vi "NEW数据采集传输系统.vi"() -> ()   [LabVIEW 2016, in "数据传输系统-02.lvlib"]
uses:
  <vilib>/Utility/miscctls.llb/LVPointTypeDef.ctl
  <vilib>/picture/picture.llb/imagedata.ctl
  <vilib>/Utility/config.llb/NI_LVConfig.lvlib
  update/update.lvlib
panel:
  in  "每日自动重发":bool
  in  "串口透传":bool
  in  "共享MN":bool
  out "剖面数据补发":bool
  out "日志信息补发":bool
  out "数据补发":bool
  in  "自动更新":bool
  in  "数据补传":bool caption="确定"
  out "数据库打开失败次数":dbl
  out "与工控通信指示灯":bool
  out "判断数据反馈":enum16{"非严格判断", "严格判断", "不判断"}(ring)
  in  "暂停上传":bool
  in  "配置表":bool caption="确定"
  in  "updateconfiguration":T1={"主机"="27.154.58.30", "用户"="update", "密码"="std23506", "远程路径"="数据传输系统\\平台数据传输系统.exe", "下载文件名"="平台数据传输系统.exe", "软件版本"=""}
  out "标题显示":string
  in  "更新":bool
  in  "系统编码选择框":string(combo)="地表水质量监测"
  out "数据发送通道":enum16{"TCP", "VISA"}(ring)
  in  "baud rate":u32=9600 caption="波特率"
  in  "VISA resource name":refnum<visa-resource-name> caption="VISA资源名称"
  in  "实时数据发送时间间隔/min":i32=1
  in  "数据组合发送":bool
  in  "2011发送":bool
  out "数据发送协议":enum16{"2005-212协议", "2017-212协议"}(ring)=enum."2017-212协议"
  in  "重发时间":T2(ring)
  in  "重发日期":T3(ring)
  in  "开机启动":bool
  in  "每周自动重发":bool=TRUE
  in  "确定":bool
  in  "返回":bool
  in  "PW":string
  in  "MN":string
  in  "PORT":string
  in  "IP":string
  in  "站点设备":string
  in  "站点名称":string
  out "设置超时时间/min":i32=1
  out "状态信息":T4={"1st Error to Convert "=63, "步骤 "=enum."发送数据", "元素"="实时数据", "TCP服务端掉线计数"=0, "TCP掉线时间节点"="2019/05/08 15:24:17"} {"1st Error to Convert" items=["无错误", "参数错误", "内存已满", "超出区域", "文件结束", "文件已打开", "一般文件IO错误", "未找到文件", "文件权限错误", "磁盘已满", "路径副本", "打开过多文件", "未启用", "未找到资源文件", "无法添加资源", "未找到资源", "未找到图像", "图像内存错误", "画笔不存在", "配置错误类型", "配置未找到解析段", "配置解析错误", "配置内存错误", "错误外部代码格式", "错误外部代码偏移量", "外部代码不存在", "空窗口", "销毁窗口错误", "空菜单", "打印已中止", "错误打印记录", "打印驱动程序错误", "打印时窗口错误", "打印时内存错误", "打印对话框错误", "一般打印错误", "无效设备引用句柄", "设备未找到", "设备参数错误", "设备单位错误", "无法打开设备", "设备调用已中止", "一般错误", "用户已取消", "对象ID过低", "对象ID过高", "对象不在堆中", "未知的堆", "错误DefProc ID", "DefProc不在表格中", "范围外信息", "空方法", "未知信息", "不支持管理器调用", "错误地址", "连接过程中", "连接超时", "连接过程中", "不支持网络属性", "网络错误", "正在使用的地址", "系统缺少内存", "连接已中止", "连接已拒绝", "连接未建立", "连接已建立", "连接已关闭", "初始化错误（交互应用程序管理器）", "错误事件发生", "等待无约束事件发生处理程序", "事件发生队列溢出", "错误路径", "未发出信号量", "未识别类型（交互应用程序管理器）"]}
  out "数据接收超时指示灯":bool
  out "空闲时间/s":string
  out "系统时间":string
  out "实时小时数据上传":bool
  out "系统状态改变":bool
  out "软件版本":string
  out "掉线指示":bool
  out "核查数据上传":bool
  out "配置信息":T5
  in  "参数配置":bool
  out "反控数据发送":bool
  out "读取报文显示":string
  out "发送报文显示":string
  out "心跳包":bool
  out "通信状态":bool
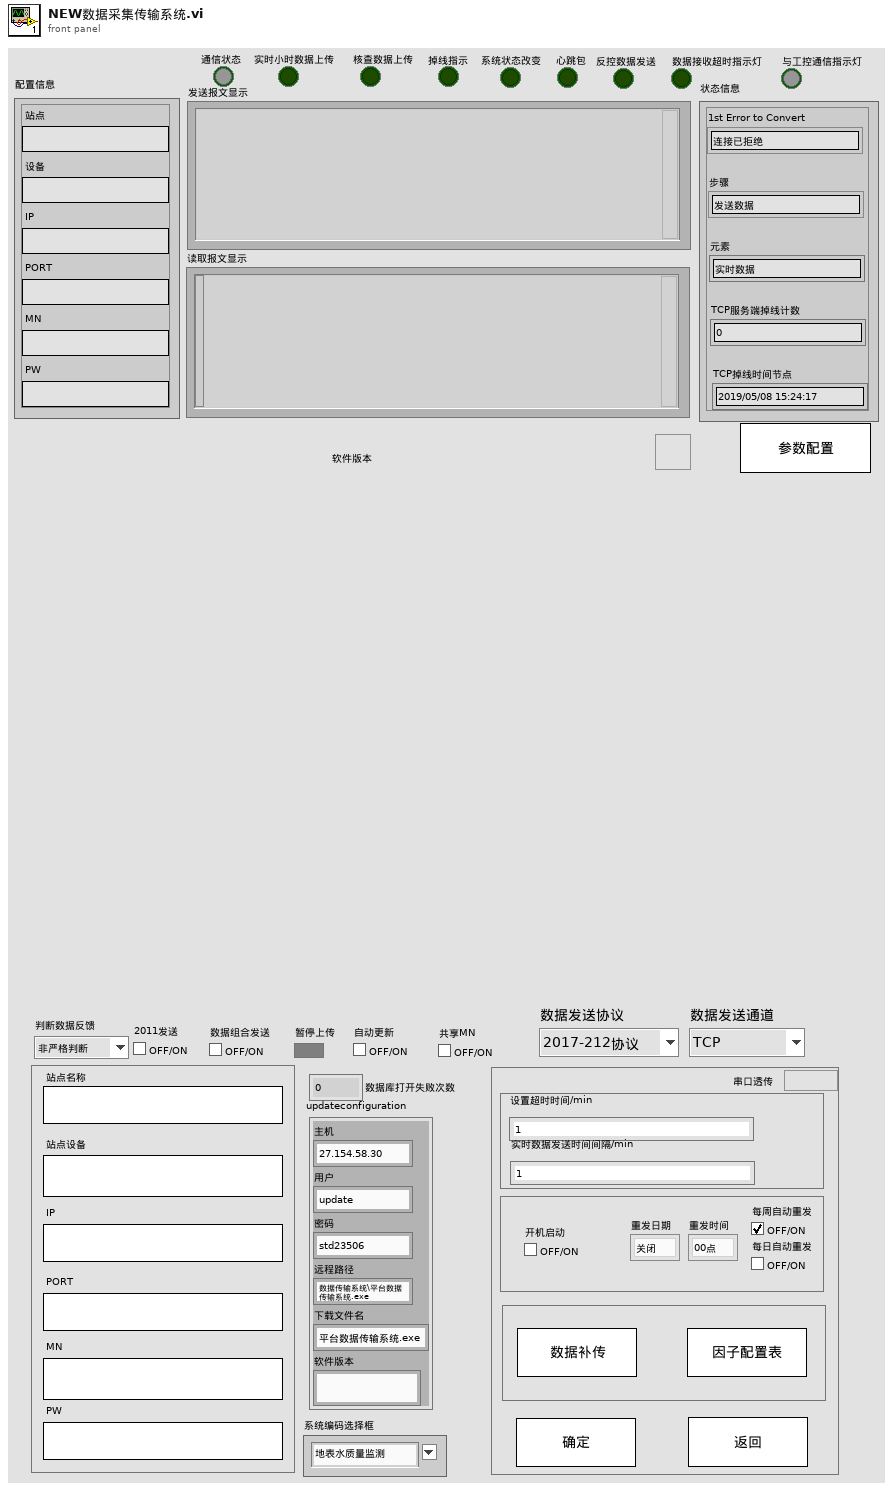
[diagram p1: front panel]
types:
  T1 = cluster{"主机":string, "用户":string, "密码":string, "远程路径":string, "下载文件名":string, "软件版本":string}
  T2 = enum16{"00点", "01点", "02点", "03点", "04点", "05点", "06点", "07点", "08点", "09点", "10点", "11点", "12点", "13点", "14点", "15点", "16点", "17点", "18点", "19点", "20点", "21点", "22点", "23点"}
  T3 = enum16{"关闭", "星期日", "星期一", "星期二", "星期三", "星期四", "星期五", "星期六"}
  T4 = cluster{"1st Error to Convert ":i32, "步骤 ":enum16{"打开连接", "发送数据", "读取数据", "数据处理", "关闭连接"}, "元素":string, "TCP服务端掉线计数":i32, "TCP掉线时间节点":string}
  T5 = cluster{"站点":string, "设备":string, "IP":string, "PORT":string, "MN":string, "PW":string}
  T6 = typedef "imagedata.ctl" = cluster{"image type":i32, "image depth":i32, "image":u8[], "mask":u8[], "colors":u32[], "Rectangle":cluster{"left":i16, "top":i16, "right":i16, "bottom":i16}}
  T7 = typedef "LVPointTypeDef.ctl" = cluster{"Horizontal":i16, "Vertical":i16}
  T8 = cluster{"setini":string, "sysini":string, "hechaini":string, "actualwrite":string, "actualread":string, "datasent":string, "反控命令信息队列":string, "反控与仪器交互":string}
  T9 = cluster{"配置表格[0]":string, "配置表格[1]":string, "配置表格[2]":string, "配置表格[3]":string, "配置表格[4]":string, "配置表格[5]":string, "配置表格[6]":string, "配置表格[7]":string, "配置表格[8]":string, "配置表格[9]":string, "配置表格[10]":string, "配置表格[11]":string, "配置表格[12]":string, "配置表格[13]":string, "配置表格[14]":string, "配置表格[15]":string, "配置表格[16]":string, "配置表格[17]":string, "配置表格[18]":string, "配置表格[19]":string, "配置表格[20]":string, "配置表格[21]":string, "配置表格[22]":string, "配置表格[23]":string, "配置表格[24]":string, "配置表格[25]":string, "配置表格[26]":string, "配置表格[27]":string, "配置表格[28]":string, "配置表格[29]":string, "配置表格[30]":string, "配置表格[31]":string, "配置表格[32]":string, "配置表格[33]":string, "配置表格[34]":string, "配置表格[35]":string, "配置表格[36]":string, "配置表格[37]":string}
  T10 = cluster{"[0]":dbl, "[1]":dbl, "[2]":dbl, "[3]":dbl, "[4]":dbl, "[5]":dbl, "[6]":dbl, "[7]":dbl, "[8]":dbl, "[9]":dbl, "[10]":dbl, "[11]":dbl, "[12]":dbl, "[13]":dbl, "[14]":dbl, "[15]":dbl, "[16]":dbl, "[17]":dbl, "[18]":dbl, "[19]":dbl, "[20]":dbl, "[21]":dbl, "[22]":dbl, "[23]":dbl, "[24]":dbl, "[25]":dbl, "[26]":dbl, "[27]":dbl, "[28]":dbl, "[29]":dbl, "[30]":dbl, "[31]":dbl, "[32]":dbl, "[33]":dbl, "[34]":dbl, "[35]":dbl, "[36]":dbl, "[37]":dbl}
  T11 = cluster{"时间标识":timestamp, "设备":string, "日志信息":string, "流程参数":string}
  T12 = typedef "NI_LVConfig.lvlib/Config Data RefNum.ctl" = refnum<k1>
  T13 = cluster{"CODMn":bool, "CODCr":bool, "DO":bool, "铜":bool, "PH":bool, "氨氮":bool, "比电导率":bool, "水温":bool, "COD":bool, "浊度":bool, "总氮":bool, "总磷":bool, "叶绿素a":bool, "藻密度":bool, "水位":bool, "流速":bool, "瞬时流量":bool, "累积流量":bool, "亚硝氮":bool, "硫化物":bool, "ORP":bool, "铅":bool, "镉":bool, "锌":bool, "镍":bool, "锰":bool, "汞":bool, "气温":bool, "气压":bool, "风速":bool, "风向":bool, "盐度":bool, "磷酸盐":bool, "硝氮":bool, "氟化物":bool, "挥发酚":bool, "氯化物":bool}
  T14 = cluster{"time1":string, "time2":string, "time3":string, "time4":string, "time5":string, "time6":string, "time7":string, "time8":string, "time9":string, "time10":string, "time11":string, "time12":string, "time13":string, "time14":string, "time15":string, "time16":string, "time17":string, "time18":string, "time19":string, "time20":string, "time21":string, "time22":string, "time23":string, "time24":string, "time25":string, "time26":string, "time27":string, "time28":string, "time29":string, "time30":string, "time31":string, "time32":string, "time33":string, "time34":string, "time35":string, "time36":string, "time37":string, "time38":string}
  T15 = cluster{"[0]":string, "[1]":string, "[2]":string, "[3]":string, "[4]":string, "[5]":string, "[6]":string, "[7]":string}
  T16 = cluster{"[0]":string, "[1]":string, "[2]":string, "[3]":string, "[4]":string, "[5]":string, "[6]":string, "[7]":string, "[8]":string, "[9]":string, "[10]":string, "[11]":string, "[12]":string, "[13]":string, "[14]":string}
  T17 = cluster{"[0]":string, "[1]":string, "[2]":string, "[3]":string, "[4]":string, "[5]":string, "[6]":string}
  T18 = cluster{"[0]":string, "[1]":string, "[2]":string, "[3]":string, "[4]":string, "[5]":string, "[6]":string, "[7]":string, "[8]":string, "[9]":string, "[10]":string, "[11]":string, "[12]":string, "[13]":string, "[14]":string, "[15]":string, "[16]":string, "[17]":string}
  T19 = cluster{"[0]":string, "[1]":string, "[2]":string, "[3]":string, "[4]":string, "[5]":string, "[6]":string, "[7]":string, "[8]":string, "[9]":string}
  T20 = cluster{"[0]":string, "[1]":string, "[2]":string, "[3]":string, "[4]":string, "[5]":string, "[6]":string, "[7]":string, "[8]":string, "[9]":string, "[10]":string, "[11]":string, "[12]":string, "[13]":string, "[14]":string, "[15]":string, "[16]":string, "[17]":string, "[18]":string, "[19]":string, "[20]":string, "[21]":string, "[22]":string, "[23]":string, "[24]":string, "[25]":string, "[26]":string, "[27]":string, "[28]":string, "[29]":string, "[30]":string, "[31]":string, "[32]":string, "[33]":string, "[34]":string, "[35]":string, "[36]":string, "[37]":string}
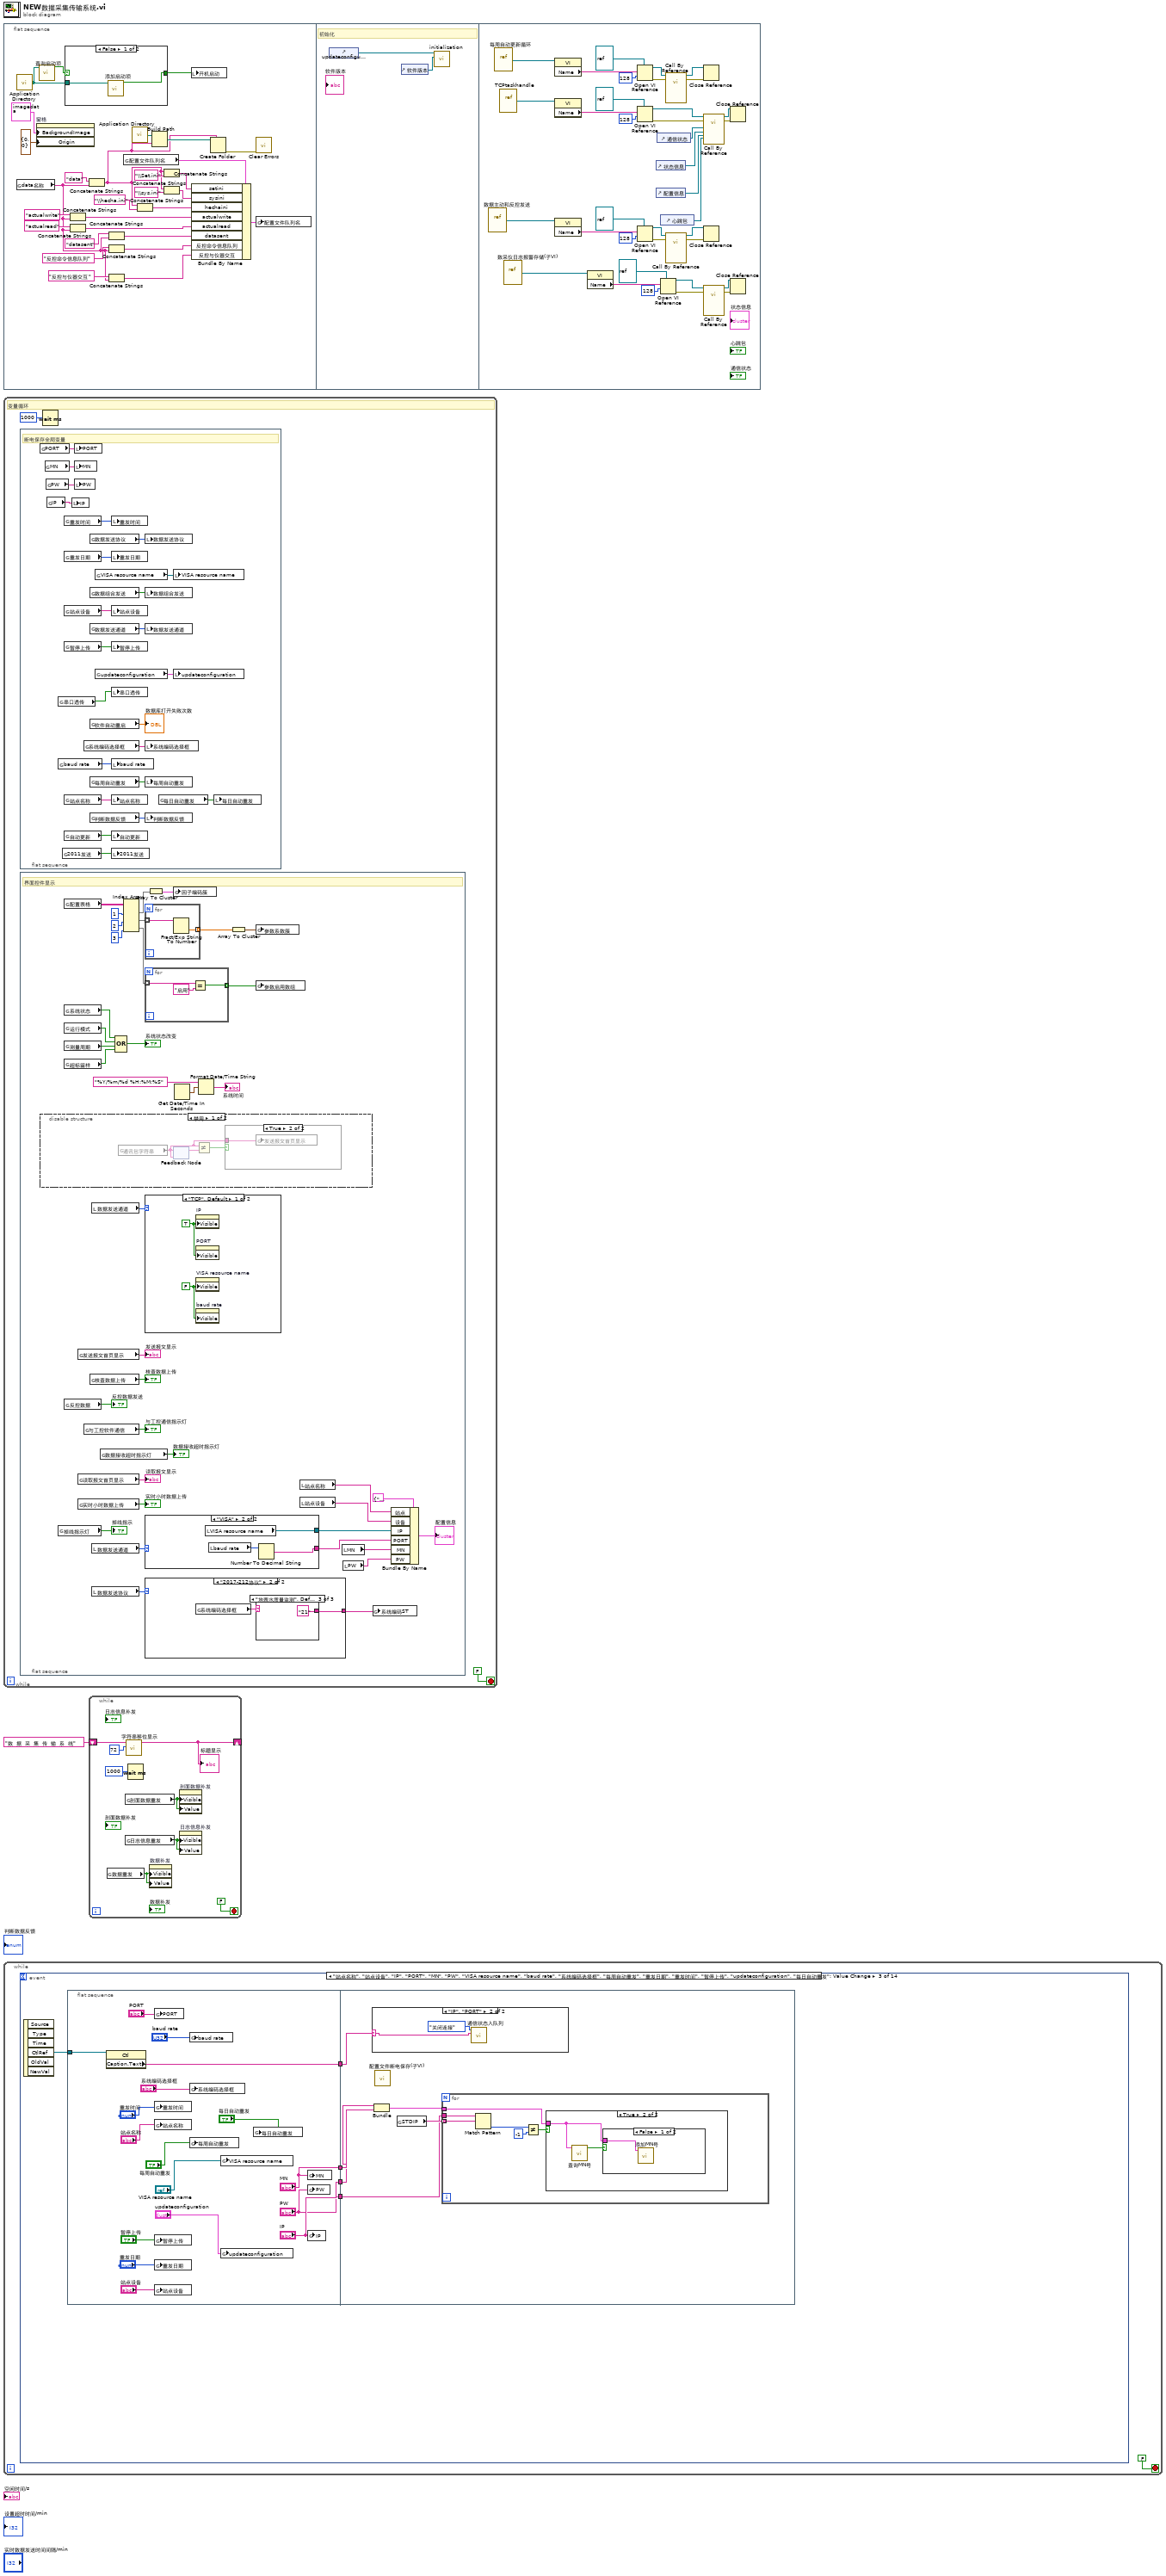
[diagram p0: block diagram]
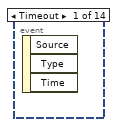
[diagram p2: hidden frame]
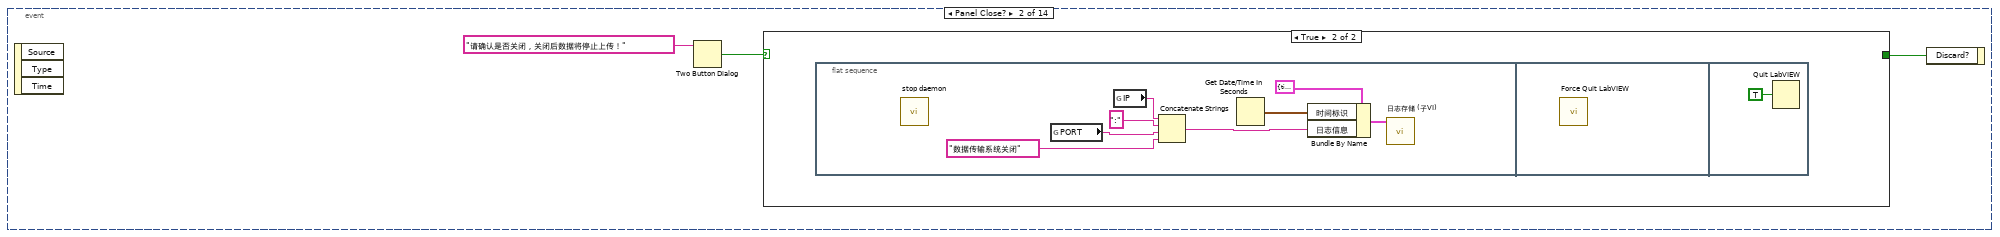
[diagram p3: hidden frame]
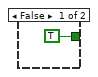
[diagram p4: hidden frame]
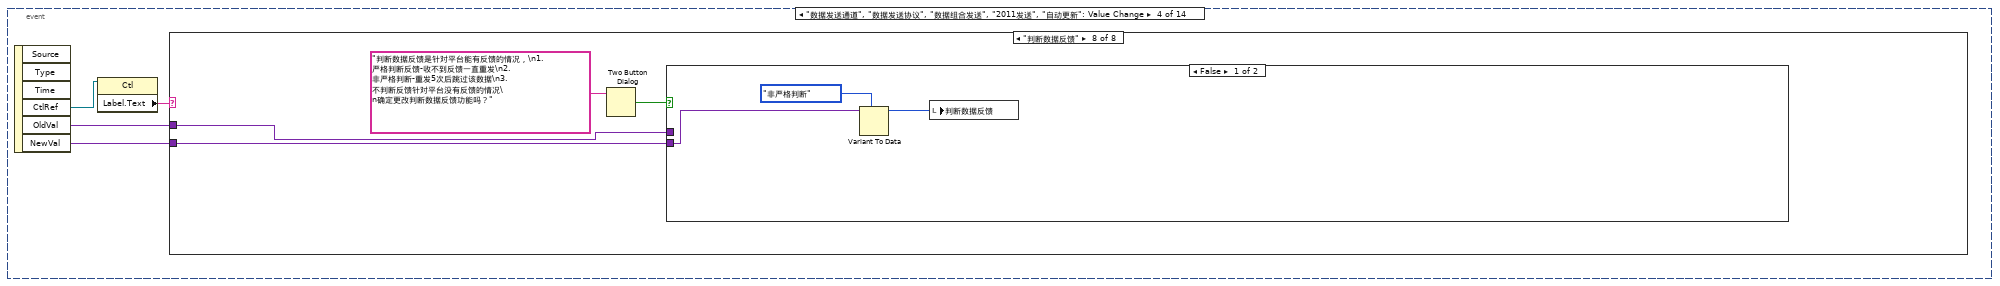
[diagram p8: hidden frame]
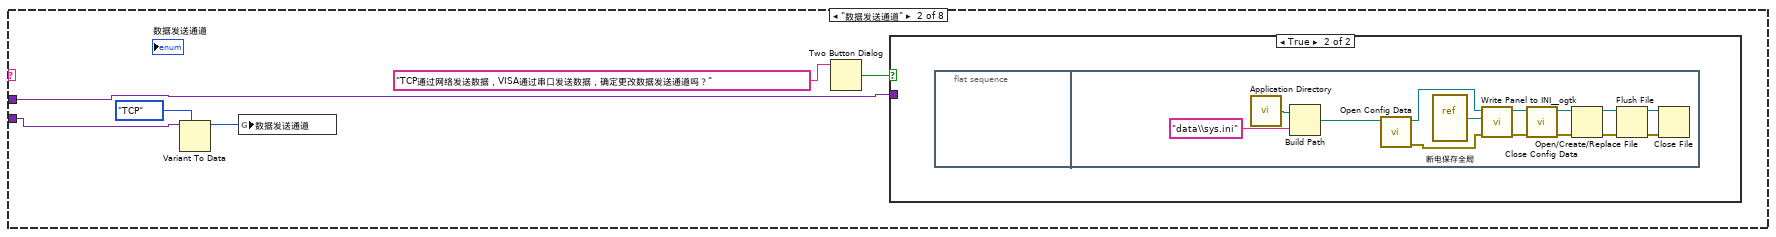
[diagram p10: hidden frame]
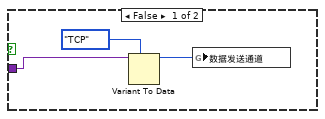
[diagram p11: hidden frame]
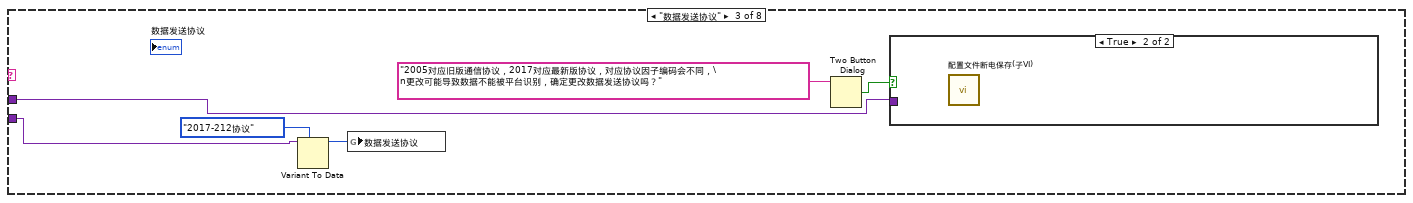
[diagram p12: hidden frame]
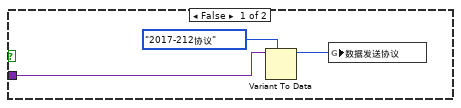
[diagram p13: hidden frame]
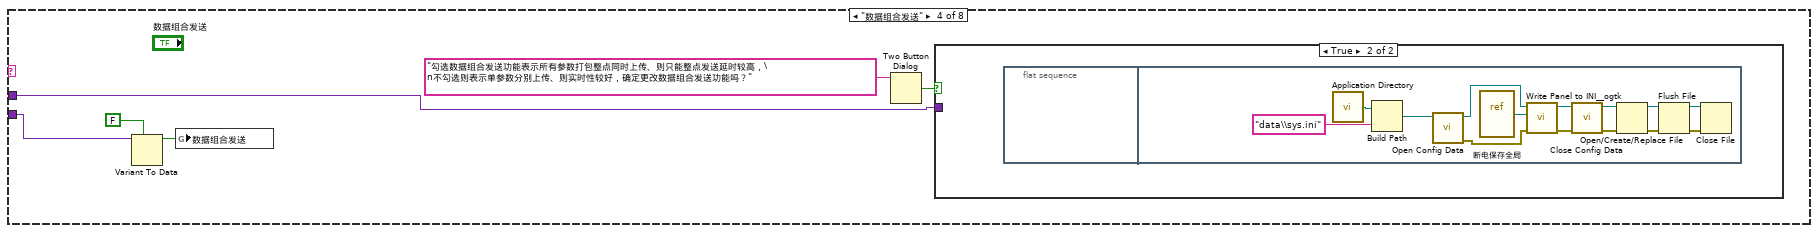
[diagram p14: hidden frame]
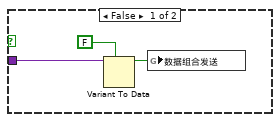
[diagram p15: hidden frame]
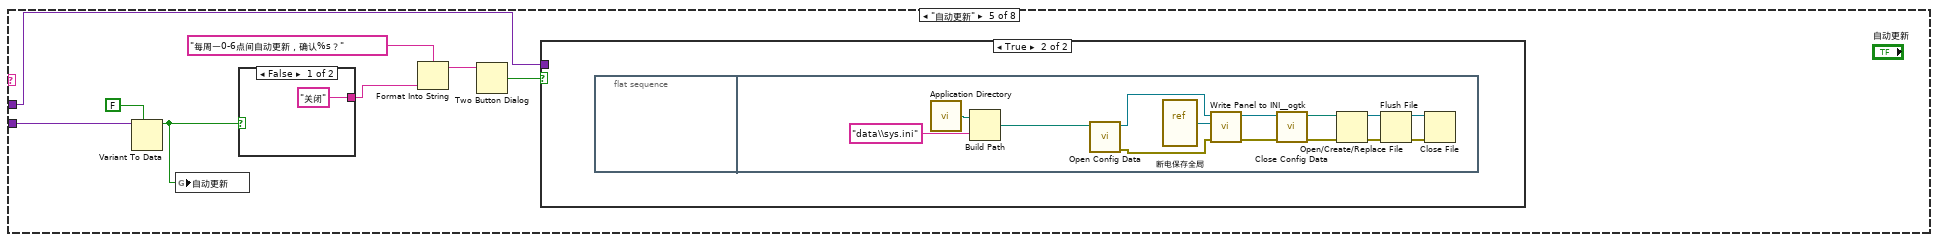
[diagram p16: hidden frame]
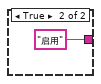
[diagram p17: hidden frame]
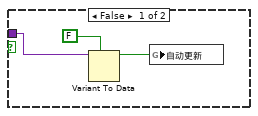
[diagram p18: hidden frame]
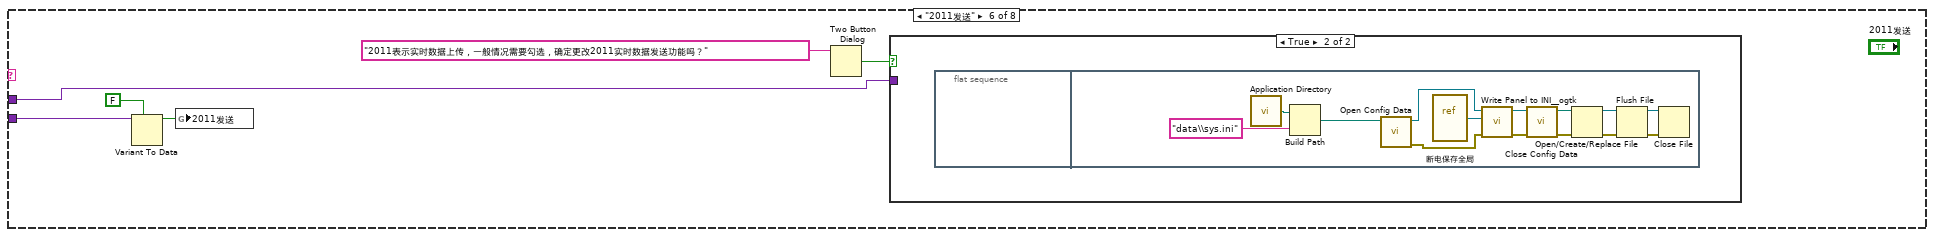
[diagram p19: hidden frame]
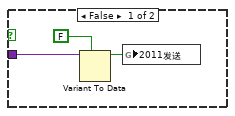
[diagram p20: hidden frame]
diagram:
  n1 = flat-sequence {
    frame #0 {
      n2 = global read "断电保存全局.vi" "data名称"() -> (w4:string)
      n3 = call <vilib>:"Application Directory.vi"() -> ("Application Directory"=w8:path)
      n4 = property on="窗格" class="Pane"("BackgroundImage"=T6 {"image type"=0, "image depth"=24, "image"=array[12288000 elements], "mask"=[], "colors"=[], "Rectangle"={"left"=0, "top"=0, "right"=2560, "bottom"=1600}} ("image data"), "Origin"=T7 {"Horizontal"=0, "Vertical"=0} ("原点")) -> ()  [unwired: 2 in, 2 out]
      n5 = call "查询启动项.vi"("启动文件路径"=w8) -> ("包含启动项"=w7:bool)  [unwired: 9 in, 1 out]
      n6 = case shown="False" w7 {
        selector: w7 -> [_ w33]
        tunnel: w8 -> [w32 _]
        tunnel: [w31 w33] -> w6
        frame False {
          n7 = call "添加启动项.vi"("启动文件路径"=w32) -> ("添加成功标记"=w31:bool)  [unwired: 9 in, 1 out]
        }
        frame True {
        }
      }
      n8 = Concatenate Strings("actualwrite" ("名称（未命名）"), w4) -> (w18:string)
      n9 = Concatenate Strings("actualread" ("名称（未命名）"), w4) -> (w16:string)
      n10 = Concatenate Strings("data" ("对话框窗口（创建文件夹）"), w4) -> (w23:string)
      n11 = Concatenate Strings("datasent" ("名称（未命名）"), w4) -> (w14:string)
      n12 = Concatenate Strings("反控命令信息队列" ("名称（未命名）"), w4) -> (w10:string)
      n13 = Concatenate Strings("反控与仪器交互" ("名称（未命名）"), w4) -> (w11:string)
      n14 = global read "全局1.vi" "配置文件队列名"() -> (w2:T8)
      n15 = call <vilib>:"Application Directory.vi"() -> ("Application Directory"=w29:path)
      n16 = Concatenate Strings(w23, "\\hecha.ini" ("名称或相对路径")) -> (w21:string)
      n17 = Build Path(base path=w29, name or relative path=w23) -> (appended path=w28:path)
      n18 = Concatenate Strings(w23, "\\Set.ini" ("名称或相对路径")) -> (w25:string)
      n19 = Concatenate Strings(w23, "\\sys.ini" ("名称或相对路径")) -> (w22:string)
      n20 = local write "开机启动"(w6) -> ()
      n21 = Bundle By Name(cluster=w2, "setini"=w25, "sysini"=w22, "hechaini"=w21, "actualwrite"=w18, "actualread"=w16, "datasent"=w14, "反控命令信息队列"=w10, "反控与仪器交互"=w11) -> (w3:T8)
      n22 = Create Folder(prompt (Create Folder)=w23, path (use dialog)=w28) -> (error out=w27:errorcluster)  [unwired: 1 in, 2 out]
      n23 = call <vilib>:"Clear Errors.vi"("error in (no error)"=w27) -> ()  [unwired: 5 in, 2 out]
      n24 = global write "全局1.vi" "配置文件队列名"(w3) -> ()
    }
    frame #1 {
      # "初始化"
      n25 = control-ref of="updateconfiguration"() -> (w35:refnum<vi>)
      n26 = control-ref of="软件版本"() -> (w34:refnum<vi>)
      n27 = call "initialization.vi"("软件版本"=w34, "updateconfiguration"=w35) -> ()  [unwired: 9 in]
    }
    frame #2 {
      n28 = vi-ref "数据主动和反控发送.vi"() -> (w63:refnum<vi>)
      n29 = vi-ref "每周自动更新循环.vi"() -> (w55:refnum<vi>)
      n30 = vi-ref "TCPtaskhandle.vi"() -> (w40:refnum<vi>)
      n31 = vi-ref "数采仪日志报警存储(子VI).vi"() -> (w64:refnum<vi>)
      n32 = property class="VI"(reference=w55) -> ("Name"=w48:string)  [unwired: 1 in, 2 out]
      n33 = property class="VI"(reference=w40) -> ("Name"=w47:string)  [unwired: 1 in, 2 out]
      n34 = property class="VI"(reference=w63) -> ("Name"=w62:string)  [unwired: 1 in, 2 out]
      n35 = property class="VI"(reference=w64) -> ("Name"=w71:string)  [unwired: 1 in, 2 out]
      n36 = Open VI Reference(type specifier VI Refnum (for type only)=refnum<vi> refnum, vi path=w48, options=128 ("选项")) -> (vi reference=w50:refnum<vi>, error out=w52:errorcluster)  [unwired: 3 in]
      n37 = Open VI Reference(type specifier VI Refnum (for type only)=refnum<vi> refnum, vi path=w47, options=128 ("选项")) -> (vi reference=w45:refnum<vi>, error out=w43:errorcluster)  [unwired: 3 in]
      n38 = Open VI Reference(type specifier VI Refnum (for type only)=refnum<vi> refnum, vi path=w62, options=128 ("选项")) -> (vi reference=w60:refnum<vi>, error out=w58:errorcluster)  [unwired: 3 in]
      n39 = control-ref of="状态信息"() -> (w38:refnum<vi>)
      n40 = control-ref of="配置信息"() -> (w37:refnum<vi>)
      n41 = control-ref of="通信状态"() -> (w39:refnum<vi>)
      n42 = control-ref of="心跳包"() -> (w36:refnum<vi>)
      n43 = Open VI Reference(type specifier VI Refnum (for type only)=refnum<vi> refnum, vi path=w71, options=128 ("选项")) -> (vi reference=w69:refnum<vi>, error out=w67:errorcluster)  [unwired: 3 in]
      n44 = call-by-ref "?"(reference=w50, error in=w52) -> (reference out=w54:refnum<vi>, error out=w53:errorcluster)  [unwired: 12 in]
      n45 = call-by-ref "?"(reference=w60, error in=w58) -> (reference out=w56:refnum<vi>, error out=w57:errorcluster)  [unwired: 12 in]
      n46 = Close Reference(reference=w54, error in (no error)=w53) -> ()  [unwired: 1 out]
      n47 = call-by-ref "?"(reference=w45, error in=w43, "心跳包"=w36, "配置信息"=w37, "状态信息"=w38, "通信状态"=w39) -> (reference out=w41:refnum<vi>, error out=w42:errorcluster)  [unwired: 8 in]
      n48 = Close Reference(reference=w56, error in (no error)=w57) -> ()  [unwired: 1 out]
      n49 = call-by-ref "?"(reference=w69, error in=w67) -> (reference out=w65:refnum<vi>, error out=w66:errorcluster)  [unwired: 12 in]
      n50 = Close Reference(reference=w41, error in (no error)=w42) -> ()  [unwired: 1 out]
      n51 = Close Reference(reference=w65, error in (no error)=w66) -> ()  [unwired: 1 out]
    }
  }
  n52 = while {
    stop <- FALSE stop-if-true
    # "变量循环"
    n53 = flat-sequence {
      frame #0 {
        # "断电保存全局变量"
        n54 = global read "断电保存全局.vi" "PORT"() -> (w160:string)
        n55 = global read "断电保存全局.vi" "MN"() -> (w159:string)
        n56 = global read "断电保存全局.vi" "PW"() -> (w158:string)
        n57 = global read "断电保存全局.vi" "IP"() -> (w161:string)
        n58 = global read "断电保存全局.vi" "串口透传"() -> (w142:bool)
        n59 = global read "断电保存全局.vi" "baud rate"() -> (w156:u32)
        n60 = global read "断电保存全局.vi" "2011发送"() -> (w152:bool)
        n61 = global read "断电保存全局.vi" "重发时间"() -> (w147:T2)
        n62 = global read "断电保存全局.vi" "重发日期"() -> (w154:T3)
        n63 = global read "断电保存全局.vi" "站点设备"() -> (w162:string)
        n64 = global read "断电保存全局.vi" "暂停上传"() -> (w146:bool)
        n65 = global read "断电保存全局.vi" "站点名称"() -> (w163:string)
        n66 = global read "断电保存全局.vi" "自动更新"() -> (w144:bool)
        n67 = local write "IP"(w161) -> ()
        n68 = local write "PORT"(w160) -> ()
        n69 = local write "MN"(w159) -> ()
        n70 = local write "PW"(w158) -> ()
        n71 = global read "断电保存全局.vi" "系统编码选择框"() -> (w148:string)
        n72 = global read "断电保存全局.vi" "数据发送协议"() -> (w150:enum16{"2005-212协议", "2017-212协议"})
        n73 = global read "断电保存全局.vi" "数据组合发送"() -> (w151:bool)
        n74 = global read "断电保存全局.vi" "数据发送通道"() -> (w149:enum16{"TCP", "VISA"})
        n75 = global read "全局1.vi" "软件自动重启"() -> (→"数据库打开失败次数":dbl)
        n76 = global read "断电保存全局.vi" "每周自动重发"() -> (w155:bool)
        n77 = global read "断电保存全局.vi" "判断数据反馈"() -> (w153:enum16{"非严格判断", "严格判断", "不判断"})
        n78 = global read "断电保存全局.vi" "VISA resource name"() -> (w157:refnum<visa-resource-name>)
        n79 = global read "断电保存全局.vi" "updateconfiguration"() -> (w143:T1)
        n80 = local write "重发时间"(w147) -> ()
        n81 = local write "重发日期"(w154) -> ()
        n82 = local write "站点设备"(w162) -> ()
        n83 = local write "暂停上传"(w146) -> ()
        n84 = local write "串口透传"(w142) -> ()
        n85 = local write "baud rate"(w156) -> ()
        n86 = local write "站点名称"(w163) -> ()
        n87 = local write "自动更新"(w144) -> ()
        n88 = local write "2011发送"(w152) -> ()
        n89 = local write "数据发送协议"(w150) -> ()
        n90 = local write "数据组合发送"(w151) -> ()
        n91 = local write "数据发送通道"(w149) -> ()
        n92 = local write "系统编码选择框"(w148) -> ()
        n93 = local write "每周自动重发"(w155) -> ()
        n94 = local write "判断数据反馈"(w153) -> ()
        n95 = global read "断电保存全局.vi" "每日自动重发"() -> (w141:bool)
        n96 = local write "VISA resource name"(w157) -> ()
        n97 = local write "updateconfiguration"(w143) -> ()
        n98 = local write "每日自动重发"(w141) -> ()
      }
    }
    n99 = flat-sequence {
      frame #0 {
        # "界面控件显示"
        n100 = disable-structure shown="禁用" {
          frame Disabled {
            n101 = global read "全局1.vi" "通讯包字符串"() -> (w114:string)
            n102 = feedback #1(w114) -> (w115:string)
            n103 = feedback-in #1(w114) -> ()
            n104 = Not Equal?(x=w114, y=w115) -> (x != y?=w113:bool)
            n105 = case shown="True" w113 {
              tunnel: w114 -> [_ w116]
              frame False {
              }
              frame True {
                n106 = global write "全局1.vi" "发送报文首页显示"(w116) -> ()
              }
            }
          }
          frame Enabled {
          }
        }
        n107 = global read "全局 数据发送重叠.vi" "掉线指示灯"() -> (→"掉线指示":bool)
        n108 = global read "断电保存全局.vi" "配置表格"() -> (w84:string[][])
        n109 = global read "全局1.vi" "系统状态"() -> (w86:bool)
        n110 = global read "全局1.vi" "运行模式"() -> (w87:bool)
        n111 = global read "全局1.vi" "测量周期"() -> (w88:bool)
        n112 = global read "全局1.vi" "超标留样"() -> (w89:bool)
        n113 = global read "全局1.vi" "反控数据"() -> (→"反控数据发送":bool)
        n114 = global read "全局1.vi" "发送报文首页显示"() -> (→"发送报文显示":string)
        n115 = global read "全局1.vi" "读取报文首页显示"() -> (→"读取报文显示":string)
        n116 = global read "全局1.vi" "实时小时数据上传"() -> (→"实时小时数据上传":bool)
        n117 = global read "全局1.vi" "与工控软件通信"() -> (→"与工控通信指示灯":bool)
        n118 = global read "全局1.vi" "核查数据上传"() -> (→"核查数据上传":bool)
        n119 = local read "数据发送通道"() -> (w94:enum16{"TCP", "VISA"})
        n120 = local read "数据发送通道"() -> (w112:enum16{"TCP", "VISA"})
        n121 = local read "数据发送协议"() -> (w101:enum16{"2005-212协议", "2017-212协议"})
        n122 = global read "全局 数据发送重叠.vi" "数据接收超时指示灯"() -> (→"数据接收超时指示灯":bool)
        n123 = Compound Arithmetic op=OR ("复合运算")(w86, w87, w88, w89) -> (→"系统状态改变":bool)
        n124 = Index Array(array=w84, index (col) #1=1 ("禁用的索引 (列)"), index (col) #2=2 ("索引 (列)"), index (col) #3=3 ("索引 (列)")) -> (element #1=w82:string[], element #2=w76:string[], element #3=w78:string[])  [unwired: 3 in]
        n125 = for {
          tunnel: w76 -> [w118] mode=indexing
          tunnel: [w117] -> w75 mode=indexing
          n126 = Fract/Exp String To Number(string=w118) -> (number=w117:dbl)  [unwired: 3 in, 1 out]
        }
        n127 = for {
          tunnel: w78 -> [w121] mode=indexing
          tunnel: [w119] -> w77 mode=indexing
          n128 = Equal?(x=w121, y="启用") -> (x = y?=w119:bool)
        }
        n129 = case shown="\"TCP\", Default" w94 {
          frame "TCP", Default {
            w122 = TRUE ("可见")
            w123 = FALSE ("可见")
            n130 = property on="IP" class="Str"("Visible"=w122) -> ()  [unwired: 2 in, 2 out]
            n131 = property on="PORT" class="Str"("Visible"=w122) -> ()  [unwired: 2 in, 2 out]
            n132 = property on="VISA resource name" class="VISAName"("Visible"=w123) -> ()  [unwired: 2 in, 2 out]
            n133 = property on="baud rate" class="DigNum (strict)"("Visible"=w123) -> ()  [unwired: 2 in, 2 out]
          }
          frame "VISA" {
            w124 = FALSE ("可见")
            w125 = TRUE ("可见")
            n134 = property on="IP" class="Str"("Visible"=w124) -> ()  [unwired: 2 in, 2 out]
            n135 = property on="PORT" class="Str"("Visible"=w124) -> ()  [unwired: 2 in, 2 out]
            n136 = property on="VISA resource name" class="VISAName"("Visible"=w125) -> ()  [unwired: 2 in, 2 out]
            n137 = property on="baud rate" class="DigNum (strict)"("Visible"=w125) -> ()  [unwired: 2 in, 2 out]
          }
        }
        n138 = case shown="\"VISA\"" w112 {
          tunnel: [w137 w140] -> w109
          tunnel: [w136 w138] -> w106
          frame "TCP", Default {
            n139 = local read "PORT"() -> (w136:string)
            n140 = local read "IP"() -> (w137:string)
          }
          frame "VISA" {
            n141 = local read "VISA resource name"() -> (w140:refnum<visa-resource-name>)
            n142 = local read "baud rate"() -> (w139:u32)
            n143 = Number To Decimal String(number=w139) -> (decimal integer string=w138:string)  [unwired: 1 in]
          }
        }
        n144 = case shown="\"2017-212协议\"" w101 {
          tunnel: [w126 w131] -> w100
          frame "2005-212协议", Default {
            n145 = global read "断电保存全局.vi" "系统编码选择框"() -> (w127:string)
            n146 = case shown="\"地表水体污染源\"" w127 {
              tunnel: ["52" ("设备编码MN") "32" ("设备编码MN") "21" ("设备编码MN")] -> w126
              frame "污水排放过程监测" {
              }
              frame "地表水体污染源" {
              }
              frame "地表水质量监测", Default {
              }
            }
          }
          frame "2017-212协议" {
            n147 = global read "断电保存全局.vi" "系统编码选择框"() -> (w132:string)
            n148 = case shown="\"地表水质量监测\", Default" w132 {
              tunnel: ["52" ("设备编码MN") "32" ("设备编码MN") "21" ("设备编码MN")] -> w131
              frame "污水排放过程监测" {
              }
              frame "地表水体污染源" {
              }
              frame "地表水质量监测", Default {
              }
            }
          }
        }
        n149 = Array To Cluster(array=w82) -> (cluster=w85:T9)
        n150 = global write "断电保存全局.vi" "因子编码簇"(w85) -> ()
        n151 = Get Date/Time In Seconds() -> (seconds since 1Jan1904=w102:timestamp)
        n152 = Format Date/Time String(time format string (%c)="%Y/%m/%d %H:%M:%S" ("时间格式字符串(%c)"), seconds (now)=w102) -> (date/time string=→"系统时间":string)  [unwired: 1 in]
        n153 = Array To Cluster(array=w75) -> (cluster=w79:T10)
        n154 = global write "断电保存全局.vi" "参数系数簇"(w79) -> ()
        n155 = global write "断电保存全局.vi" "参数启用数组"(w77) -> ()
        n156 = local read "站点名称"() -> (w108:string)
        n157 = local read "站点设备"() -> (w107:string)
        n158 = local read "MN"() -> (w105:string)
        n159 = local read "PW"() -> (w104:string)
        n160 = global write "全局1.vi" "系统编码ST"(w100) -> ()
        n161 = Bundle By Name(cluster=T5 {"站点"="", "设备"="", "IP"="", "PORT"="", "MN"="", "PW"=""} ("配置信息"), "站点"=w108, "设备"=w107, "IP"=w109, "PORT"=w106, "MN"=w105, "PW"=w104) -> (→"配置信息":T5)
      }
    }
    n162 = Wait (ms)(milliseconds to wait=u32 1000 ("等待时间（毫秒）")) -> ()  [unwired: 1 out]
  }
  n163 = while {
    stop <- FALSE stop-if-true
    n164 = event shown="[2] \"站点名称\", \"站点设备\", \"IP\", \"PORT\", \"MN\", \"PW\", \"VISA resource name\", \"baud rate\", \"系统编码选择框\", \"每周自动重发\", \"重发日期\", \"重发时间\", \"暂停上传\", \"updateconfiguration\", \"每日自动重发\": Value Change" {
      selector: _ -> [_ _ _ _ _ _ _ _ _ _ _ _ _ _]
      dyn-events: _ -> [_ _ _ _ _ _ _ _ _ _ _ _ _ _]
      timeout: _ -> [_ _ _ _ _ _ _ _ _ _ _ _ _ _]
      event Timeout {
        n165 = event-data() -> ()  [unwired: 1 in, 3 out]
      }
      event Panel Close? {
        n166 = event-data() -> ()  [unwired: 1 in, 3 out]
        n167 = Two Button Dialog(message="请确认是否关闭，关闭后数据将停止上传！" ("消息")) -> (T button?=w166:bool)  [unwired: 2 in]
        n168 = case shown="True" w166 {
          tunnel: [TRUE _] -> w165
          frame False {
          }
          frame True {
            n169 = flat-sequence {
              frame #0 {
                n170 = call "stop daemon.vi"() -> ()  [unwired: 11 in, 1 out]
                n171 = global read "断电保存全局.vi" "PORT"() -> (w172:string)
                n172 = global read "断电保存全局.vi" "IP"() -> (w174:string)
                n173 = Concatenate Strings(w174, ":", w172, "数据传输系统关闭" ("日志信息")) -> (w170:string)
                n174 = Get Date/Time In Seconds() -> (seconds since 1Jan1904=w176:timestamp)
                n175 = Bundle By Name(cluster=T11 {"时间标识"=timestamp(0 s since 1904-01-01), "设备"="数采仪", "日志信息"="", "流程参数"=""} ("data in"), "时间标识"=w176, "日志信息"=w170) -> (w175:T11)
                n176 = call "日志存储 (子VI).vi"("data in"=w175) -> ()  [unwired: 11 in]
              }
              frame #1 {
                n177 = call "Force Quit LabVIEW.vi"() -> ()  [unwired: 10 in, 2 out]
              }
              frame #2 {
                n178 = Quit LabVIEW(quit? (T)=TRUE ("退出？(T)")) -> ()
              }
            }
          }
        }
        n179 = event-data("Discard?"=w165) -> ()  [unwired: 1 in, 1 out]
      }
      event "站点名称", "站点设备", "IP", "PORT", "MN", "PW", "VISA resource name", "baud rate", "系统编码选择框", "每周自动重发", "重发日期", "重发时间", "暂停上传", "updateconfiguration", "每日自动重发": Value Change {
        n180 = event-data() -> ("CtlRef"=w182:refnum<vi>)  [unwired: 1 in, 5 out]
        n181 = flat-sequence {
          tunnel: w182 -> [w189]
          tunnel: [w188] -> w181
          tunnel: ["IP"] -> w180
          tunnel: ["MN"] -> w179
          tunnel: ["PW"] -> w178
          tunnel: w181 -> [w205]
          tunnel: w180 -> [w203]
          tunnel: w179 -> [w202]
          tunnel: w178 -> [w201]
          frame #0 {
            n182 = property class="Ctl"(reference=w189) -> ("Caption.Text"=w188:string)  [unwired: 1 in, 2 out]
            n183 = global write "断电保存全局.vi" "PORT"("PORT") -> ()
            n184 = global write "断电保存全局.vi" "重发时间"("重发时间") -> ()
            n185 = global write "断电保存全局.vi" "站点名称"("站点名称") -> ()
            n186 = global write "断电保存全局.vi" "暂停上传"("暂停上传") -> ()
            n187 = global write "断电保存全局.vi" "重发日期"("重发日期") -> ()
            n188 = global write "断电保存全局.vi" "站点设备"("站点设备") -> ()
            n189 = global write "断电保存全局.vi" "baud rate"("baud rate") -> ()
            n190 = global write "断电保存全局.vi" "系统编码选择框"("系统编码选择框") -> ()
            n191 = global write "断电保存全局.vi" "每周自动重发"("每周自动重发") -> ()
            n192 = global write "断电保存全局.vi" "VISA resource name"("VISA resource name") -> ()
            n193 = global write "断电保存全局.vi" "updateconfiguration"("updateconfiguration") -> ()
            n194 = global write "断电保存全局.vi" "每日自动重发"("每日自动重发") -> ()
            n195 = global write "断电保存全局.vi" "MN"("MN") -> ()
            n196 = global write "断电保存全局.vi" "PW"("PW") -> ()
            n197 = global write "断电保存全局.vi" "IP"("IP") -> ()
          }
          frame #1 {
            n198 = case shown="\"IP\", \"PORT\"" w205 {
              selector: w205 -> [_ w215]
              frame "假", Default {
              }
              frame "IP", "PORT" {
                n199 = call "通信状态入队列.vi"("发送报文"=w215, "枚举"=enum16{"打开连接", "发送数据", "读取数据", "数据处理", "关闭连接"}."关闭连接") -> ()  [unwired: 9 in, 1 out]
              }
            }
            n200 = Bundle("MN"=w202, "PW"=w201) -> (w200:cluster{"MN":string, "PW":string})  [unwired: 1 in]
            n201 = call "配置文件断电保存(子VI).vi"() -> ()  [unwired: 12 in]
            n202 = global read "断电保存全局.vi" "STDIP"() -> (w204:string[])
            n203 = for {
              tunnel: w204 -> [w211] mode=indexing
              tunnel: w203 -> [w210]
              tunnel: w200 -> [w206]
              n204 = Match Pattern(string=w210, regular expression=w211) -> (offset past match=w209:i32)  [unwired: 1 in, 3 out]
              n205 = Not Equal?(x=w209, y=-1) -> (x != y?=w207:bool)
              n206 = case shown="True" w207 {
                tunnel: w206 -> [_ w213]
                frame False {
                }
                frame True {
                  n207 = call "查询MN号.vi"("簇"=w213) -> ("包含启动项"=w212:bool)  [unwired: 9 in, 1 out]
                  n208 = case shown="False" w212 {
                    tunnel: w213 -> [w214 _]
                    frame False {
                      n209 = call "添加MN号.vi"("簇"=w214) -> ()  [unwired: 9 in, 2 out]
                    }
                    frame True {
                    }
                  }
                }
              }
            }
          }
        }
      }
      event "数据发送通道", "数据发送协议", "数据组合发送", "2011发送", "自动更新": Value Change {
        n210 = event-data() -> ("CtlRef"=w220:refnum<vi>, "OldVal"=w218:variant, "NewVal"=w217:variant)  [unwired: 1 in, 3 out]
        n211 = property class="Ctl"(reference=w220) -> ("Label.Text"=w219:string)  [unwired: 1 in, 2 out]
        n212 = case shown="\"判断数据反馈\"" w219 {
          tunnel: w218 -> [_ w224 w247 w256 w282 w306 w329 w350]
          tunnel: w217 -> [_ w221 w244 w253 w280 w303 w326 w349]
          frame "假", Default {
          }
          frame "数据发送通道" {
            n213 = Variant To Data(type=enum16{"TCP", "VISA"}."TCP" ("数据发送通道"), Variant=w221) -> (data=w222:enum16{"TCP", "VISA"})  [unwired: 1 in, 1 out]
            n214 = global write "断电保存全局.vi" "数据发送通道"(w222) -> ()
            n215 = Two Button Dialog(message="TCP通过网络发送数据，VISA通过串口发送数据，确定更改数据发送通道吗？" ("消息")) -> (T button?=w225:bool)  [unwired: 2 in]
            n216 = case shown="True" w225 {
              tunnel: w224 -> [w228 _]
              frame False {
                n217 = Variant To Data(type=enum16{"TCP", "VISA"}."TCP" ("数据发送通道"), Variant=w228) -> (data=w227:enum16{"TCP", "VISA"})  [unwired: 1 in, 1 out]
                n218 = global write "断电保存全局.vi" "数据发送通道"(w227) -> ()
              }
              frame True {
                n219 = flat-sequence {
                  frame #0 {
                  }
                  frame #1 {
                    n220 = call <vilib>:"Application Directory.vi"() -> ("Application Directory"=w230:path)
                    n221 = Build Path(base path=w230, name or relative path="data\\sys.ini" ("名称或相对路径")) -> (appended path=w232:path)
                    n222 = call <vilib>:"Open Config Data.vi"("configuration file path"=w232) -> ("error out"=w236:errorcluster, "refnum"=w233:T12)  [unwired: 8 in, 1 out]
                    n223 = vi-ref "断电保存全局.vi"() -> (w234:refnum<vi>)
                    n224 = call <userlib>:"Write Panel to INI__ogtk.vi"("error in (no error)"=w236, "VI ref"=w234, "refnum"=w233) -> ("error out"=w237:errorcluster, "refnum out"=w235:T12)  [unwired: 7 in]
                    n225 = call <vilib>:"Close Config Data.vi"("error in (no error)"=w237, "refnum"=w235) -> ("error out"=w242:errorcluster, "file path"=w243:path)  [unwired: 8 in]
                    n226 = Open/Create/Replace File(file path (use dialog)=w243, error in=w242) -> (refnum out=w239:refnum<file>, error out=w238:errorcluster)  [unwired: 4 in, 1 out]
                    n227 = Flush File(refnum=w239, error in=w238) -> (refnum out=w240:refnum<file>, error out=w241:errorcluster)
                    n228 = Close File(refnum=w240, error in=w241) -> ()  [unwired: 2 out]
                  }
                }
              }
            }
          }
          frame "数据发送协议" {
            n229 = Variant To Data(type=enum16{"2005-212协议", "2017-212协议"}."2017-212协议" ("数据"), Variant=w244) -> (data=w245:enum16{"2005-212协议", "2017-212协议"})  [unwired: 1 in, 1 out]
            n230 = global write "断电保存全局.vi" "数据发送协议"(w245) -> ()
            n231 = Two Button Dialog(message="2005对应旧版通信协议，2017对应最新版协议，对应协议因子编码会不同，\n更改可能导致数据不能被平台识别，确定更改数据发送协议吗？" ("消息")) -> (T button?=w248:bool)  [unwired: 2 in]
            n232 = case shown="True" w248 {
              tunnel: w247 -> [w252 _]
              frame False {
                n233 = Variant To Data(type=enum16{"2005-212协议", "2017-212协议"}."2017-212协议" ("数据"), Variant=w252) -> (data=w250:enum16{"2005-212协议", "2017-212协议"})  [unwired: 1 in, 1 out]
                n234 = global write "断电保存全局.vi" "数据发送协议"(w250) -> ()
              }
              frame True {
                n235 = call "配置文件断电保存(子VI).vi"() -> ()  [unwired: 12 in]
              }
            }
          }
          frame "数据组合发送" {
            n236 = Variant To Data(type=FALSE, Variant=w253) -> (data=w254:bool)  [unwired: 1 in, 1 out]
            n237 = global write "断电保存全局.vi" "数据组合发送"(w254) -> ()
            n238 = Two Button Dialog(message="勾选数据组合发送功能表示所有参数打包整点同时上传、则只能整点发送延时较高，\n不勾选则表示单参数分别上传、则实时性较好，确定更改数据组合发送功能吗？" ("消息")) -> (T button?=w257:bool)  [unwired: 2 in]
            n239 = case shown="True" w257 {
              tunnel: w256 -> [w260 _]
              frame False {
                n240 = Variant To Data(type=FALSE, Variant=w260) -> (data=w259:bool)  [unwired: 1 in, 1 out]
                n241 = global write "断电保存全局.vi" "数据组合发送"(w259) -> ()
              }
              frame True {
                n242 = flat-sequence {
                  frame #0 {
                  }
                  frame #1 {
                    n243 = call <vilib>:"Application Directory.vi"() -> ("Application Directory"=w262:path)
                    n244 = Build Path(base path=w262, name or relative path="data\\sys.ini" ("名称或相对路径")) -> (appended path=w264:path)
                    n245 = call <vilib>:"Open Config Data.vi"("configuration file path"=w264) -> ("error out"=w268:errorcluster, "refnum"=w265:T12)  [unwired: 8 in, 1 out]
                    n246 = vi-ref "断电保存全局.vi"() -> (w266:refnum<vi>)
                    n247 = call <userlib>:"Write Panel to INI__ogtk.vi"("error in (no error)"=w268, "VI ref"=w266, "refnum"=w265) -> ("error out"=w269:errorcluster, "refnum out"=w267:T12)  [unwired: 7 in]
                    n248 = call <vilib>:"Close Config Data.vi"("error in (no error)"=w269, "refnum"=w267) -> ("error out"=w274:errorcluster, "file path"=w275:path)  [unwired: 8 in]
                    n249 = Open/Create/Replace File(file path (use dialog)=w275, error in=w274) -> (refnum out=w271:refnum<file>, error out=w270:errorcluster)  [unwired: 4 in, 1 out]
                    n250 = Flush File(refnum=w271, error in=w270) -> (refnum out=w272:refnum<file>, error out=w273:errorcluster)
                    n251 = Close File(refnum=w272, error in=w273) -> ()  [unwired: 2 out]
                  }
                }
              }
            }
          }
          frame "自动更新" {
            n252 = Variant To Data(type=FALSE, Variant=w280) -> (data=w278:bool)  [unwired: 1 in, 1 out]
            n253 = global write "断电保存全局.vi" "自动更新"(w278) -> ()
            n254 = case shown="False" w278 {
              tunnel: ["关闭" "启用"] -> w277
              frame False {
              }
              frame True {
              }
            }
            n255 = Format Into String(format string="每周一0-6点间自动更新，确认%s？" ("消息"), w277) -> (resulting string=w276:string)  [unwired: 2 in, 1 out]
            n256 = Two Button Dialog(message=w276) -> (T button?=w283:bool)  [unwired: 2 in]
            n257 = case shown="True" w283 {
              tunnel: w282 -> [w287 _]
              frame False {
                n258 = Variant To Data(type=FALSE, Variant=w287) -> (data=w286:bool)  [unwired: 1 in, 1 out]
                n259 = global write "断电保存全局.vi" "自动更新"(w286) -> ()
              }
              frame True {
                n260 = flat-sequence {
                  frame #0 {
                  }
                  frame #1 {
                    n261 = call <vilib>:"Application Directory.vi"() -> ("Application Directory"=w289:path)
                    n262 = Build Path(base path=w289, name or relative path="data\\sys.ini" ("名称或相对路径")) -> (appended path=w291:path)
                    n263 = call <vilib>:"Open Config Data.vi"("configuration file path"=w291) -> ("error out"=w295:errorcluster, "refnum"=w292:T12)  [unwired: 8 in, 1 out]
                    n264 = vi-ref "断电保存全局.vi"() -> (w293:refnum<vi>)
                    n265 = call <userlib>:"Write Panel to INI__ogtk.vi"("error in (no error)"=w295, "VI ref"=w293, "refnum"=w292) -> ("error out"=w296:errorcluster, "refnum out"=w294:T12)  [unwired: 7 in]
                    n266 = call <vilib>:"Close Config Data.vi"("error in (no error)"=w296, "refnum"=w294) -> ("error out"=w301:errorcluster, "file path"=w302:path)  [unwired: 8 in]
                    n267 = Open/Create/Replace File(file path (use dialog)=w302, error in=w301) -> (refnum out=w298:refnum<file>, error out=w297:errorcluster)  [unwired: 4 in, 1 out]
                    n268 = Flush File(refnum=w298, error in=w297) -> (refnum out=w299:refnum<file>, error out=w300:errorcluster)
                    n269 = Close File(refnum=w299, error in=w300) -> ()  [unwired: 2 out]
                  }
                }
              }
            }
          }
          frame "2011发送" {
            n270 = Variant To Data(type=FALSE, Variant=w303) -> (data=w304:bool)  [unwired: 1 in, 1 out]
            n271 = global write "断电保存全局.vi" "2011发送"(w304) -> ()
            n272 = Two Button Dialog(message="2011表示实时数据上传，一般情况需要勾选，确定更改2011实时数据发送功能吗？" ("消息")) -> (T button?=w307:bool)  [unwired: 2 in]
            n273 = case shown="True" w307 {
              tunnel: w306 -> [w310 _]
              frame False {
                n274 = Variant To Data(type=FALSE, Variant=w310) -> (data=w309:bool)  [unwired: 1 in, 1 out]
                n275 = global write "断电保存全局.vi" "2011发送"(w309) -> ()
              }
              frame True {
                n276 = flat-sequence {
                  frame #0 {
                  }
                  frame #1 {
                    n277 = call <vilib>:"Application Directory.vi"() -> ("Application Directory"=w312:path)
                    n278 = Build Path(base path=w312, name or relative path="data\\sys.ini" ("名称或相对路径")) -> (appended path=w314:path)
                    n279 = call <vilib>:"Open Config Data.vi"("configuration file path"=w314) -> ("error out"=w318:errorcluster, "refnum"=w315:T12)  [unwired: 8 in, 1 out]
                    n280 = vi-ref "断电保存全局.vi"() -> (w316:refnum<vi>)
                    n281 = call <userlib>:"Write Panel to INI__ogtk.vi"("error in (no error)"=w318, "VI ref"=w316, "refnum"=w315) -> ("error out"=w319:errorcluster, "refnum out"=w317:T12)  [unwired: 7 in]
                    n282 = call <vilib>:"Close Config Data.vi"("error in (no error)"=w319, "refnum"=w317) -> ("error out"=w324:errorcluster, "file path"=w325:path)  [unwired: 8 in]
                    n283 = Open/Create/Replace File(file path (use dialog)=w325, error in=w324) -> (refnum out=w321:refnum<file>, error out=w320:errorcluster)  [unwired: 4 in, 1 out]
                    n284 = Flush File(refnum=w321, error in=w320) -> (refnum out=w322:refnum<file>, error out=w323:errorcluster)
                    n285 = Close File(refnum=w322, error in=w323) -> ()  [unwired: 2 out]
                  }
                }
              }
            }
          }
          frame "日志、参数发送" {
            n286 = Variant To Data(type=FALSE, Variant=w326) -> (data=w327:bool)  [unwired: 1 in, 1 out]
            n287 = global write "断电保存全局.vi" "日志、参数发送"(w327) -> ()
            n288 = Two Button Dialog(message="选择是否需要仪器日志、状态和告警信息上传，一般情况需要勾选，确定更改日志、参数发送功能吗？" ("消息")) -> (T button?=w330:bool)  [unwired: 2 in]
            n289 = case shown="False" w330 {
              tunnel: w329 -> [w333 _]
              frame False {
                n290 = Variant To Data(type=FALSE, Variant=w333) -> (data=w332:bool)  [unwired: 1 in, 1 out]
                n291 = global write "断电保存全局.vi" "日志、参数发送"(w332) -> ()
              }
              frame True {
                n292 = flat-sequence {
                  frame #0 {
                  }
                  frame #1 {
                    n293 = call <vilib>:"Application Directory.vi"() -> ("Application Directory"=w335:path)
                    n294 = Build Path(base path=w335, name or relative path="data\\sys.ini" ("名称或相对路径")) -> (appended path=w337:path)
                    n295 = call <vilib>:"Open Config Data.vi"("configuration file path"=w337) -> ("error out"=w341:errorcluster, "refnum"=w338:T12)  [unwired: 8 in, 1 out]
                    n296 = vi-ref "断电保存全局.vi"() -> (w339:refnum<vi>)
                    n297 = call <userlib>:"Write Panel to INI__ogtk.vi"("error in (no error)"=w341, "VI ref"=w339, "refnum"=w338) -> ("error out"=w342:errorcluster, "refnum out"=w340:T12)  [unwired: 7 in]
                    n298 = call <vilib>:"Close Config Data.vi"("error in (no error)"=w342, "refnum"=w340) -> ("error out"=w347:errorcluster, "file path"=w348:path)  [unwired: 8 in]
                    n299 = Open/Create/Replace File(file path (use dialog)=w348, error in=w347) -> (refnum out=w344:refnum<file>, error out=w343:errorcluster)  [unwired: 4 in, 1 out]
                    n300 = Flush File(refnum=w344, error in=w343) -> (refnum out=w345:refnum<file>, error out=w346:errorcluster)
                    n301 = Close File(refnum=w345, error in=w346) -> ()  [unwired: 2 out]
                  }
                }
              }
            }
          }
          frame "判断数据反馈" {
            n302 = Two Button Dialog(message="判断数据反馈是针对平台能有反馈的情况，\n1.严格判断反馈-收不到反馈一直重发\n2.非严格判断-重发5次后跳过该数据\n3.不判断反馈针对平台没有反馈的情况\n确定更改判断数据反馈功能吗？" ("消息")) -> (T button?=w351:bool)  [unwired: 2 in]
            n303 = case shown="False" w351 {
              tunnel: w350 -> [_ _]
              tunnel: w349 -> [w354 w356]
              frame False {
                n304 = Variant To Data(type=enum16{"非严格判断", "严格判断", "不判断"}."非严格判断" ("判断数据反馈"), Variant=w354) -> (data=w353:enum16{"非严格判断", "严格判断", "不判断"})  [unwired: 1 in, 1 out]
                n305 = local write "判断数据反馈"(w353) -> ()
              }
              frame True {
                n306 = flat-sequence {
                  tunnel: w356 -> [w357]
                  frame #0 {
                    n307 = Variant To Data(type=enum16{"非严格判断", "严格判断", "不判断"}."非严格判断" ("判断数据反馈"), Variant=w357) -> (data=w359:enum16{"非严格判断", "严格判断", "不判断"})  [unwired: 1 in, 1 out]
                    n308 = global write "断电保存全局.vi" "判断数据反馈"(w359) -> ()
                  }
                  frame #1 {
                    n309 = call <vilib>:"Application Directory.vi"() -> ("Application Directory"=w360:path)
                    n310 = Build Path(base path=w360, name or relative path="data\\sys.ini" ("名称或相对路径")) -> (appended path=w362:path)
                    n311 = call <vilib>:"Open Config Data.vi"("configuration file path"=w362) -> ("error out"=w366:errorcluster, "refnum"=w363:T12)  [unwired: 8 in, 1 out]
                    n312 = vi-ref "断电保存全局.vi"() -> (w364:refnum<vi>)
                    n313 = call <userlib>:"Write Panel to INI__ogtk.vi"("error in (no error)"=w366, "VI ref"=w364, "refnum"=w363) -> ("error out"=w367:errorcluster, "refnum out"=w365:T12)  [unwired: 7 in]
                    n314 = call <vilib>:"Close Config Data.vi"("error in (no error)"=w367, "refnum"=w365) -> ("error out"=w372:errorcluster, "file path"=w373:path)  [unwired: 8 in]
                    n315 = Open/Create/Replace File(file path (use dialog)=w373, error in=w372) -> (refnum out=w369:refnum<file>, error out=w368:errorcluster)  [unwired: 4 in, 1 out]
                    n316 = Flush File(refnum=w369, error in=w368) -> (refnum out=w370:refnum<file>, error out=w371:errorcluster)
                    n317 = Close File(refnum=w370, error in=w371) -> ()  [unwired: 2 out]
                  }
                }
              }
            }
          }
        }
      }
      event "确定": Value Change {
        n318 = event-data() -> ()  [unwired: 1 in, 6 out]
        n319 = call "通信状态入队列.vi"("枚举"=enum16{"打开连接", "发送数据", "读取数据", "数据处理", "关闭连接"}."关闭连接") -> ()  [unwired: 10 in, 1 out]
      }
      event "配置表": Value Change {
        n320 = event-data() -> ()  [unwired: 1 in, 6 out]
        n321 = call "参数配置表.vi"() -> ()  [unwired: 12 in]
      }
      event "串口透传": Value Change {
        n322 = event-data() -> ()  [unwired: 1 in, 6 out]
        n323 = flat-sequence {
          frame #0 {
            n324 = global write "断电保存全局.vi" "串口透传"("串口透传") -> ()
          }
          frame #1 {
            n325 = call "配置文件断电保存(子VI).vi"() -> ()  [unwired: 12 in]
          }
        }
        n326 = call "串口配置.vi"() -> ()  [unwired: 12 in]
      }
      event "参数配置": Value Change {
        n327 = event-data() -> ()  [unwired: 1 in, 6 out]
        n328 = local read "MN"() -> (w380:string)
        n329 = local read "PW"() -> (w379:string)
        n330 = property on="窗格" class="Pane"("Origin"=T7 {"Horizontal"=0, "Vertical"=1000} ("原点")) -> ()  [unwired: 2 in, 2 out]
        n331 = call <vilib>:"Application Directory.vi"() -> ("Application Directory"=w382:path)
        n332 = Bundle("MN"=w380, "PW"=w379) -> (w378:cluster{"MN":string, "PW":string})  [unwired: 1 in]
        n333 = call "查询启动项.vi"("启动文件路径"=w382) -> ("error out"=w377:errorcluster, "包含启动项"=w381:bool)  [unwired: 9 in]
        n334 = local write "开机启动"(w381) -> ()
        n335 = call "查询MN号.vi"("error in (no error)"=w377, "簇"=w378) -> ("包含启动项"=w376:bool)  [unwired: 8 in, 1 out]
        n336 = local write "共享MN"(w376) -> ()
      }
      event "返回": Value Change {
        n337 = event-data() -> ()  [unwired: 1 in, 6 out]
        n338 = property on="窗格" class="Pane"("Origin"=T7 {"Horizontal"=0, "Vertical"=0} ("原点")) -> ()  [unwired: 2 in, 2 out]
      }
      event "数据补传": Value Change {
        n339 = event-data() -> ()  [unwired: 1 in, 6 out]
        n340 = global read "全局1.vi" "数据发送起始时间"() -> (w387:timestamp)
        n341 = call "数据补传对话框.vi"("起始时间"=w387) -> ("参数数值out"=w386:T13, "结束时间输出"=w388:timestamp, "起始时间输出"=w389:timestamp, "输出"=w390:bool, "只补小时数据输出"=w385:bool)  [unwired: 6 in]
        n342 = case shown="True" w390 {
          tunnel: w389 -> [_ w399]
          tunnel: w388 -> [_ w400]
          tunnel: w386 -> [_ w396]
          tunnel: w385 -> [_ w398]
          frame False {
          }
          frame True {
            w397 = TRUE ("数据重发")
            n343 = global write "全局1.vi" "数据发送起始时间"(w399) -> ()
            n344 = global write "断电保存全局.vi" "数据重发结束时间"(w400) -> ()
            n345 = Cluster To Array(cluster=w396) -> (array=w394:bool[])
            n346 = global read "全局 水样时间.vi" "水样数据索引"() -> (w395:T14)
            n347 = Format Date/Time String(time format string (%c)="%Y/%m/%d %H:%M:%S" ("时间格式字符串(%c)"), seconds (now)=w399) -> (date/time string=w392:string)  [unwired: 1 in]
            n348 = Cluster To Array(cluster=w395) -> (array=w393:string[])
            n349 = global write "断电保存全局.vi" "数据重发"(w397) -> ()
            n350 = case shown="False" w398 {
              tunnel: w392 -> [w414 _]
              tunnel: w397 -> [w407 _]
              frame False {
                n351 = global write "断电保存全局.vi" "日志信息重发"(w407) -> ()
                n352 = global write "断电保存全局.vi" "剖面数据重发"(w407) -> ()
                n353 = global write "全局 水样时间.vi" "剖面多参数数据时间"(w414) -> ()
                n354 = global write "全局 水样时间.vi" "剖面数据时间"(w414) -> ()
                n355 = global write "断电保存全局.vi" "数据重发时间戳"(w414) -> ()
                n356 = Initialize Array(w414, 8 ("维数大小")) -> (w410:string[])
                n357 = Initialize Array(w414, 15 ("维数大小")) -> (w411:string[])
                n358 = Array To Cluster(array=w410) -> (cluster=w409:T15)
                n359 = global read "断电保存全局.vi" "数据组合发送"() -> (w415:bool)
                n360 = global write "全局 时间2.vi" "仪器日志索引"(w409) -> ()
                n361 = Array To Cluster(array=w411) -> (cluster=w412:T16)
                n362 = case shown="False" w415 {
                  tunnel: w414 -> [w416 _]
                  frame False {
                    n363 = global write "全局 时间2.vi" "标样核查索引起始时间"(w416) -> ()
                    n364 = global write "全局 时间2.vi" "加标回收索引起始时间"(w416) -> ()
                    n365 = global write "全局 时间2.vi" "跨度核查索引起始时间"(w416) -> ()
                    n366 = global write "全局 时间2.vi" "3092日志索引起始时间"(w416) -> ()
                    n367 = global write "全局 时间2.vi" "零点核查索引起始时间"(w416) -> ()
                    n368 = Initialize Array(w416, 7 ("维数大小")) -> (w420:string[])
                    n369 = Initialize Array(w416, 8 ("维数大小")) -> (w419:string[])
                    n370 = Initialize Array(w416, 18 ("维数大小")) -> (w423:string[])
                    n371 = Initialize Array(w416, 10 ("维数大小")) -> (w428:string[])
                    n372 = Array To Cluster(array=w419) -> (cluster=w418:T15)
                    n373 = Array To Cluster(array=w420) -> (cluster=w421:T17)
                    n374 = global write "全局 时间2.vi" "平行样索引"(w421) -> ()
                    n375 = global write "全局 时间2.vi" "加标回收索引"(w421) -> ()
                    n376 = global write "全局 时间2.vi" "仪器日志索引"(w418) -> ()
                    n377 = Array To Cluster(array=w423) -> (cluster=w424:T18)
                    n378 = Array To Cluster(array=w428) -> (cluster=w427:T19)
                    n379 = global write "全局 时间2.vi" "标样核查索引"(w424) -> ()
                    n380 = global write "全局 时间2.vi" "集成干预索引"(w424) -> ()
                    n381 = global write "全局 时间2.vi" "跨度核查索引"(w427) -> ()
                    n382 = global write "全局 时间2.vi" "零点核查索引"(w427) -> ()
                  }
                  frame True {
                  }
                }
                n383 = global write "全局 时间2.vi" "仪器参数索引"(w412) -> ()
              }
              frame True {
                n384 = global write "断电保存全局.vi" "2011发送"(FALSE ("2011发送")) -> ()
              }
            }
            n385 = for {
              tunnel: w394 -> [w406] mode=indexing
              tunnel: w393 -> [w404] mode=indexing
              tunnel: w392 -> [w405]
              tunnel: [w403] -> w391 mode=indexing
              n386 = Select(t=w405, s=w406, f=w404) -> (s? t:f=w403:string)
            }
            n387 = Array To Cluster(array=w391) -> (cluster=w401:T20)
            n388 = global write "全局 水样时间.vi" "水样数据索引"(w401) -> ()
          }
        }
      }
      event "开机启动": Value Change {
        n389 = event-data() -> ("CtlRef"=w431:refnum<vi>, "OldVal"=w430:bool, "NewVal"=w432:bool)  [unwired: 1 in, 3 out]
        n390 = case shown="False" w432 {
          tunnel: w431 -> [w434 w447]
          tunnel: w430 -> [w433 w446]
          frame False {
            n391 = Two Button Dialog(message="是否删除开机启动？" ("消息"), 1:"否" ("F按钮名称（“取消”）"), 2:"是" ("T按钮名称（“确定”）")) -> (T button?=w435:bool)
            n392 = case shown="True" w435 {
              tunnel: w434 -> [w440 _]
              tunnel: w433 -> [w439 _]
              frame False {
                n393 = property class="Bool (strict)"(reference=w440, "Value"=w439) -> ()  [unwired: 1 in, 2 out]
              }
              frame True {
                n394 = call <vilib>:"Application Directory.vi"() -> ("Application Directory"=w442:path)
                n395 = call "删除启动项.vi"("启动文件路径"=w442) -> ("删除标记"=w441:bool)  [unwired: 9 in, 1 out]
                n396 = case shown="True" w441 {
                  tunnel: ["删除开机启动失败" ("T按钮名称（“确定”）") "删除开机启动成功" ("T按钮名称（“确定”）")] -> w443
                  frame False {
                  }
                  frame True {
                  }
                }
                n397 = One Button Dialog(message=w443) -> ()  [unwired: 1 in, 1 out]
              }
            }
          }
          frame True {
            n398 = Two Button Dialog(message="是否添加开机启动？" ("消息"), 1:"否" ("F按钮名称（“取消”）"), 2:"是" ("T按钮名称（“确定”）")) -> (T button?=w448:bool)
            n399 = case shown="True" w448 {
              tunnel: w447 -> [w453 _]
              tunnel: w446 -> [w452 _]
              frame False {
                n400 = property class="Bool (strict)"(reference=w453, "Value"=w452) -> ()  [unwired: 1 in, 2 out]
              }
              frame True {
                n401 = call <vilib>:"Application Directory.vi"() -> ("Application Directory"=w456:path)
                n402 = call "添加启动项.vi"("启动文件路径"=w456) -> ("添加成功标记"=w455:bool)  [unwired: 9 in, 1 out]
                n403 = case shown="True" w455 {
                  tunnel: ["添加开机启动失败" ("T按钮名称（“确定”）") "添加开机启动成功" ("T按钮名称（“确定”）")] -> w454
                  frame False {
                  }
                  frame True {
                  }
                }
                n404 = One Button Dialog(message=w454) -> ()  [unwired: 1 in, 1 out]
              }
            }
          }
        }
      }
      event "共享MN": Value Change {
        n405 = event-data() -> ("CtlRef"=w460:refnum<vi>, "OldVal"=w459:bool, "NewVal"=w461:bool)  [unwired: 1 in, 3 out]
        n406 = case shown="True" w461 {
          tunnel: w460 -> [w463 w478]
          tunnel: w459 -> [w462 w477]
          frame False {
            n407 = Two Button Dialog(message="是否取消该MN号共享？" ("消息"), 1:"否" ("F按钮名称（“取消”）"), 2:"是" ("T按钮名称（“确定”）")) -> (T button?=w464:bool)
            n408 = case shown="True" w464 {
              tunnel: w463 -> [w469 _]
              tunnel: w462 -> [w468 _]
              frame False {
                n409 = property class="Bool (strict)"(reference=w469, "Value"=w468) -> ()  [unwired: 1 in, 2 out]
              }
              frame True {
                n410 = local read "MN"() -> (w473:string)
                n411 = local read "PW"() -> (w472:string)
                n412 = Bundle("MN"=w473, "PW"=w472) -> (w471:cluster{"MN":string, "PW":string})  [unwired: 1 in]
                n413 = call "删除MN号.vi"("簇"=w471) -> ("删除标记"=w470:bool)  [unwired: 9 in, 1 out]
                n414 = case shown="True" w470 {
                  tunnel: ["取消该MN号共享失败" ("T按钮名称（“确定”）") "取消该MN号共享成功" ("T按钮名称（“确定”）")] -> w474
                  frame False {
                  }
                  frame True {
                  }
                }
                n415 = One Button Dialog(message=w474) -> ()  [unwired: 1 in, 1 out]
              }
            }
          }
          frame True {
            n416 = Two Button Dialog(message="是否添加该MN号共享？" ("消息"), 1:"否" ("F按钮名称（“取消”）"), 2:"是" ("T按钮名称（“确定”）")) -> (T button?=w479:bool)
            n417 = case shown="True" w479 {
              tunnel: w478 -> [w484 _]
              tunnel: w477 -> [w483 _]
              frame False {
                n418 = property class="Bool (strict)"(reference=w484, "Value"=w483) -> ()  [unwired: 1 in, 2 out]
              }
              frame True {
                n419 = local read "MN"() -> (w488:string)
                n420 = local read "PW"() -> (w487:string)
                n421 = Bundle("MN"=w488, "PW"=w487) -> (w486:cluster{"MN":string, "PW":string})  [unwired: 1 in]
                n422 = call "添加MN号.vi"("簇"=w486) -> ("添加成功标记"=w485:bool)  [unwired: 9 in, 1 out]
                n423 = case shown="False" w485 {
                  tunnel: ["添加该MN号共享失败" ("T按钮名称（“确定”）") "添加该MN号共享成功" ("T按钮名称（“确定”）")] -> w489
                  frame False {
                  }
                  frame True {
                  }
                }
                n424 = One Button Dialog(message=w489) -> ()  [unwired: 1 in, 1 out]
              }
            }
          }
        }
      }
      event "更新": Value Change {
        n425 = event-data() -> ()  [unwired: 1 in, 6 out]
        n426 = call "自定义双按钮对话框.vi"("消息"="选择是否从服务器获取最新版本信息？") -> ("正式版/测试版输出"=w492:bool, "输出"=w493:bool)  [unwired: 9 in]
        n427 = case shown="True" w493 {
          tunnel: w492 -> [_ w497]
          frame False {
          }
          frame True {
            # "获取最新版本"
            n428 = local read "updateconfiguration"() -> (w502:T1)
            n429 = Unbundle By Name(w502) -> ("远程路径"=w496:string)
            n430 = case shown="True" w497 {
              tunnel: w496 -> [w503 w504]
              tunnel: [w503 w505] -> w500
              frame False {
                # "正式版"
              }
              frame True {
                # "测试版"
                n431 = String To Path(string=w504) -> (path=w506:path)
                n432 = Strip Path(path=w506) -> (name=w509:string)  [unwired: 1 out]
                n433 = Search and Replace String(input string=w504, search string=w509, replace string="beta/" ("字符串")) -> (result string=w508:string)  [unwired: 5 in, 3 out]
                n434 = Concatenate Strings(w508, w509) -> (w505:string)
              }
            }
            n435 = Search and Replace String(replace all?=TRUE ("替换全部？(F)"), input string=w500, search string="\\" ("替换字符串(\"\")"), replace string="/" ("分隔符(Tab)")) -> (result string=w495:string)  [unwired: 4 in, 3 out]
            n436 = call "Updateinter.vi"("更新包远端地址"=w495, "测试版？"=w497) -> ()  [unwired: 10 in]
          }
        }
      }
      event "IP", "PORT": Mouse Down {
        n437 = event-data() -> ("CtlRef"=w518:refnum<vi>)  [unwired: 1 in, 7 out]
        n438 = property class="Str"(reference=w518) -> (reference out=w516:refnum<vi>, "Value"=w517:string)  [unwired: 1 in, 1 out]
        n439 = call "IP键盘.vi"("OldNumber"=w517) -> ("NewNumber"=w513:string)
        n440 = String Length(string=w513) -> (length=w515:i32)
        n441 = Less Or Equal?(x=w515, y=50) -> (x <= y?=w512:bool)
        n442 = case shown="False" w512 {
          tunnel: w516 -> [w519 w523]
          tunnel: w513 -> [_ w522]
          tunnel: [w519 w523] -> w511
          tunnel: ["127.0.0.1" w522] -> w510
          frame False {
            n443 = One Button Dialog(message="超过ipv4最大长度限制,请重新输入!" ("消息")) -> ()  [unwired: 1 in, 1 out]
          }
          frame True {
          }
        }
        n444 = property class="Str"(reference=w511, "Val(Sgnl)"=w510) -> ()  [unwired: 1 in, 2 out]
      }
    }
  }
  n445 = while {
    shift-right: [w528] -> _
    shift-left: "数  据  采  集  传  输  系  统" ("标题显示") -> [w529]
    stop <- FALSE stop-if-true
    n446 = global read "断电保存全局.vi" "数据重发"() -> (w526:bool)
    n447 = global read "断电保存全局.vi" "剖面数据重发"() -> (w524:bool)
    n448 = global read "断电保存全局.vi" "日志信息重发"() -> (w525:bool)
    n449 = call "字符串移位显示.vi"("字符框大小"=72, "字符串输入"=w529) -> ("移位后字符串"=w528:string)  [unwired: 8 in, 1 out]
    "标题显示" <- w528
    n450 = Wait (ms)(milliseconds to wait=u32 1000 ("等待时间（毫秒）")) -> ()  [unwired: 1 out]
    n451 = property on="数据补发" class="Bool (strict)"("Visible"=w526, "Value"=w526) -> ()  [unwired: 2 in, 2 out]
    n452 = property on="剖面数据补发" class="Bool (strict)"("Visible"=w524, "Value"=w524) -> ()  [unwired: 2 in, 2 out]
    n453 = property on="日志信息补发" class="Bool (strict)"("Visible"=w525, "Value"=w525) -> ()  [unwired: 2 in, 2 out]
  }
